vi "updateiqual.vi"   [LabVIEW 2012]
uses:
  <vilib>/addons/database/Auxilliary.llb/DB Tools Parameter Dir.ctl
  <vilib>/addons/database/Auxilliary.llb/DB Tools DataTypes.ctl
  resultShow.vi
  <vilib>/addons/database/NI_Database_API.lvlib
types:
  T1 = cluster{"takesTime":refnum<vi>, "userStatus":refnum<vi>, "userName":refnum<vi>, "connectionMode":refnum<vi>, "productsName":refnum<vi>, "rigStatus":refnum<vi>, "总成扫码":refnum<vi>}
  T2 = typedef "NI_Database_API.lvlib/DB Tools DataTypes.ctl" = enum16{"String", "Long (I32)", "Single (SGL)", "Double (DBL)", "Date/Time", "Binary"}
  T3 = typedef "NI_Database_API.lvlib/DB Tools Parameter Dir.ctl" = enum32{"Input", "Output", "Input/Output", "Return Value"}
  T4 = cluster{"parameter name":string, "type":T2, "direction":T3, "Value":string}
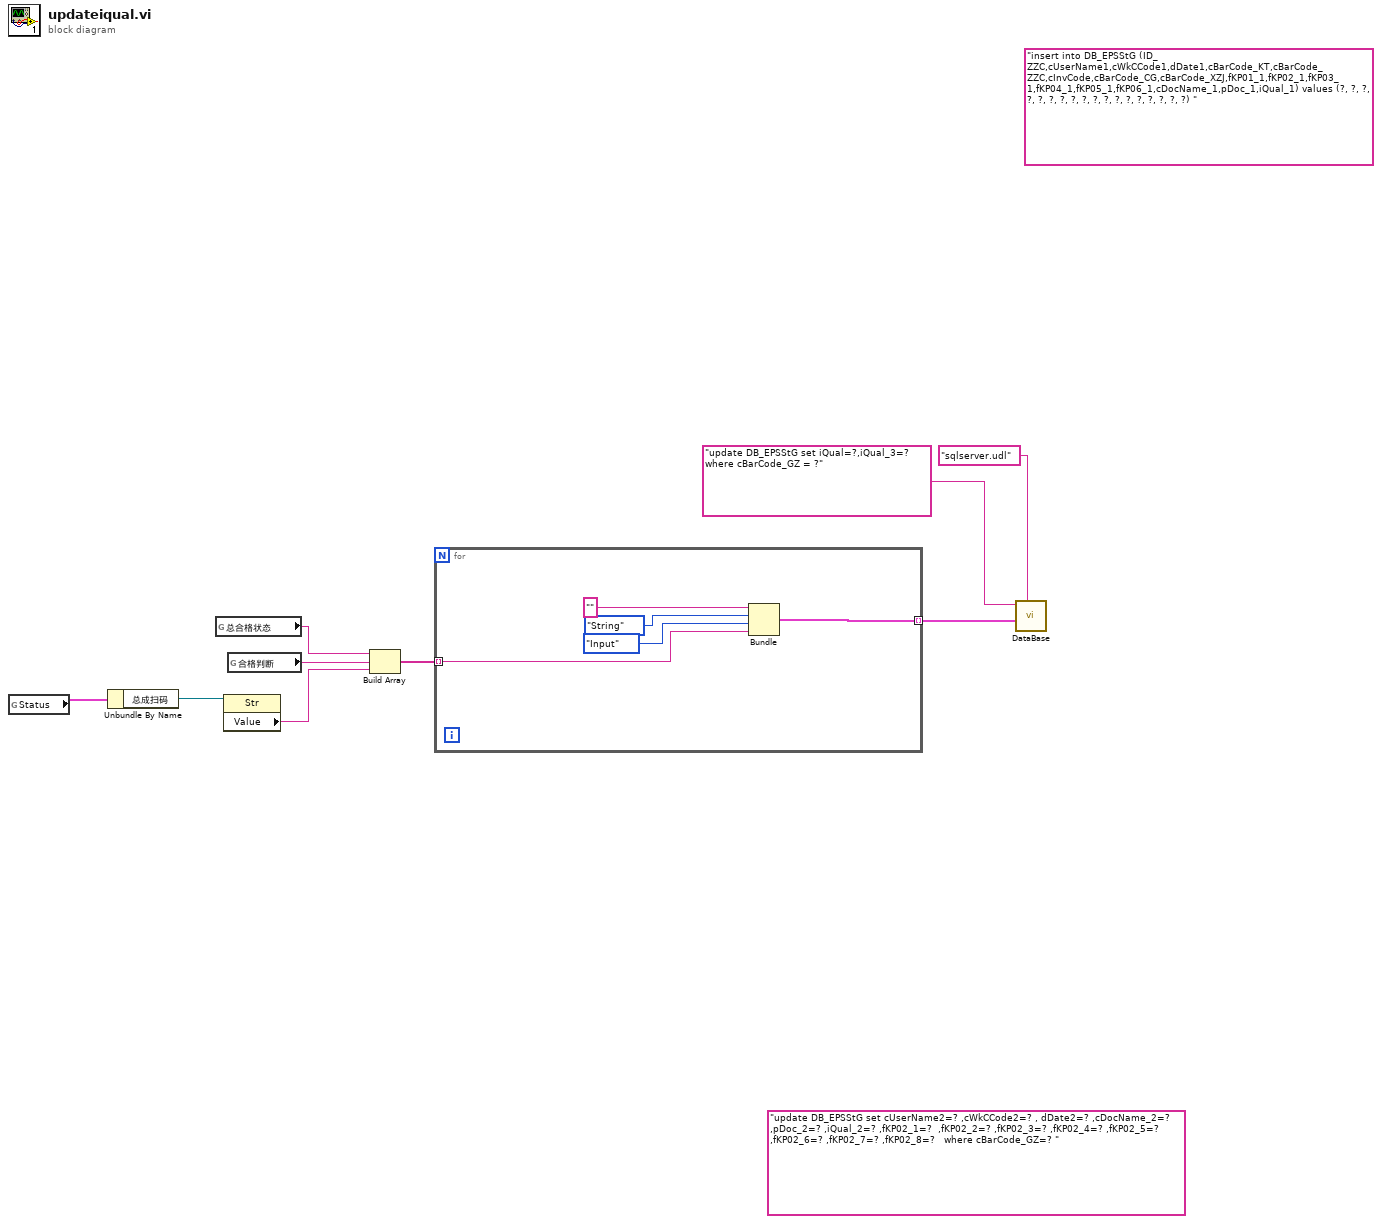
[diagram p0: block diagram]
diagram:
  (unwired) "insert into DB_EPSStG (ID_ZZC,cUserName1,cWkCCode1,dDate1,cBarCode_KT,cBarCode_ZZC,cInvCode,cBarCode_CG,cBarCode_XZJ,fKP01_1,fKP02_1,fKP03_1,fKP04_1,fKP05_1,fKP06_1,cDocName_1,pDoc_1,iQual_1) values (?, ?, ?, ?, ?, ?, ?, ?, ?, ?, ?, ?, ?, ?, ?, ?, ?, ?) " ("SQL query")
  (unwired) "update DB_EPSStG set cUserName2=? ,cWkCCode2=? , dDate2=? ,cDocName_2=? ,pDoc_2=? ,iQual_2=? ,fKP02_1=?  ,fKP02_2=? ,fKP02_3=? ,fKP02_4=? ,fKP02_5=? ,fKP02_6=? ,fKP02_7=? ,fKP02_8=?   where cBarCode_GZ=? " ("SQL query")
  n1 = global read "resultShow.vi" "Status"() -> (w5:T1)
  n2 = Unbundle By Name(w5) -> ("总成扫码"=w4:refnum<vi>)
  n3 = global read "全局 3.vi" "总合格状态"() -> (w7:string)
  n4 = property class="Str"(reference=w4) -> ("Value"=w3:string)  [unwired: 1 in, 2 out]
  n5 = global read "全局 3.vi" "合格判断"() -> (w6:string)
  n6 = Build Array(w7, w6, w3) -> (w2:string[])
  n7 = for {
    tunnel: w2 -> [w11] mode=indexing
    tunnel: [w10] -> w1 mode=indexing
    n8 = Bundle("parameter name"="", "type"=DB_Tools_DataTypes."String", "direction"=DB_Tools_Parameter_Dir."Input", "Value"=w11) -> (w10:T4)  [unwired: 1 in]
  }
  n9 = call "DataBase.vi"("udl名称"="sqlserver.udl", "parameters"=w1, "SQL query"="update DB_EPSStG set iQual=?,iQual_3=? where cBarCode_GZ = ?") -> ()  [unwired: 8 in, 1 out]
